vi "13.4.2 AutoROI.vi"(8 "ErrI":errorcluster) -> (0 "ErrO":errorcluster)   [LabVIEW 2016]
uses:
  <vilib>/vision/Image Controls.llb/IMAQ Image.ctl
  <vilib>/vision/Measure.llb/Edge Options.ctl
  <vilib>/vision/Measure.llb/Edge Polarity.ctl
  <vilib>/vision/NI_Vision_Development_Module.lvlib
panel:
  out "Coordinate System":T1 {"Measurement System"."Axis Reference" items=["Direct", "Indirect"]; "Measurement System"."Angle (deg)" format="%.2f"; "Measurement System"."Origin"."Y" format="%.2f"; "Measurement System"."Origin"."X" format="%.2f"; "Reference System"."Axis Reference" items=["Direct", "Indirect"]; "Reference System"."Angle (deg)" format="%.2f"; "Reference System"."Origin"."Y" format="%.2f"; "Reference System"."Origin"."X" format="%.2f"}
  out "Distance":sgl format="%.2f"
  out "Image":T2(plugin-control)
  in  "Next":bool
  in  "Exit":bool
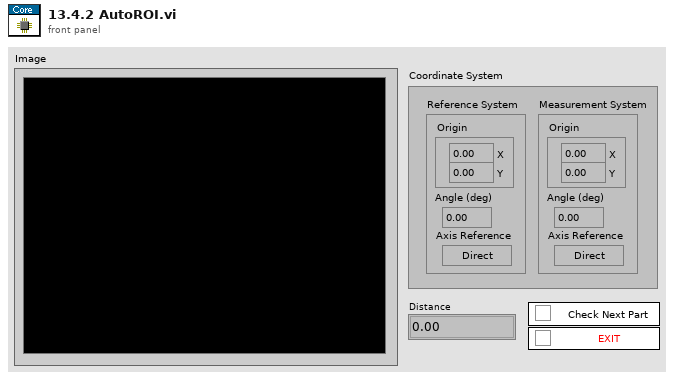
[diagram p1: front panel]
types:
  T1 = typedef "IMAQ Coordinate System" = cluster{"Reference System":cluster{"Origin":cluster{"X":sgl, "Y":sgl}, "Angle (deg)":sgl, "Axis Reference":u32}, "Measurement System":cluster{"Origin":cluster{"X":sgl, "Y":sgl}, "Angle (deg)":sgl, "Axis Reference":u32}}
  T2 = typedef "IMAQ Image.ctl" = refnum<image>
  T3 = typedef "IMAQ Rectangle" = cluster{"Left":i32, "Top":i32, "Right":i32, "Bottom":i32, "Rotation":dbl}
  T4 = cluster{"Contrast":i32, "Filter width":i32, "Steepness":i32, "Subsampling Ratio":u32, "Show Search Area":bool, "Show Search Lines":bool, "Show Edges Found":bool, "Show Result":bool}
  T5 = cluster{"Src":T2, "Dst":T2, "Parts":string[], "RefCoord":T1, "MsrCoord":T1, "MsrROI":T3}
  T6 = typedef "Edge Options.ctl" = cluster{"Edge Polarity":T7, "Kernel Size":u32, "Width":u32, "Minimum Edge Strength":sgl, "Interpolation Type":enum32{"Zero Order", "Bilinear", "Quadratic", "Cubic", "Bilinear Fixed"}, "Data Processing Method":enum32{"Average", "Median"}}
  T7 = typedef "Edge Polarity.ctl" = u32
  T8 = cluster{"Direction":u16, "Edge Options":T6, "Show Search Area":bool, "Show Search Lines":bool, "Show Edges Found":bool, "Show Result":bool, "Search Area Color":u32, "Search Lines Color":u32, "Edge Locations Color":u32, "Result Color":u32, "Overlay Group Name":string}
  T9 = typedef "ROI Descriptor" = cluster{"Global Rectangle":i32[], "Contours":cluster{"ID":enum32{"External", "Internal"}, "Type":u32, "Coordinates":i32[]}[]}
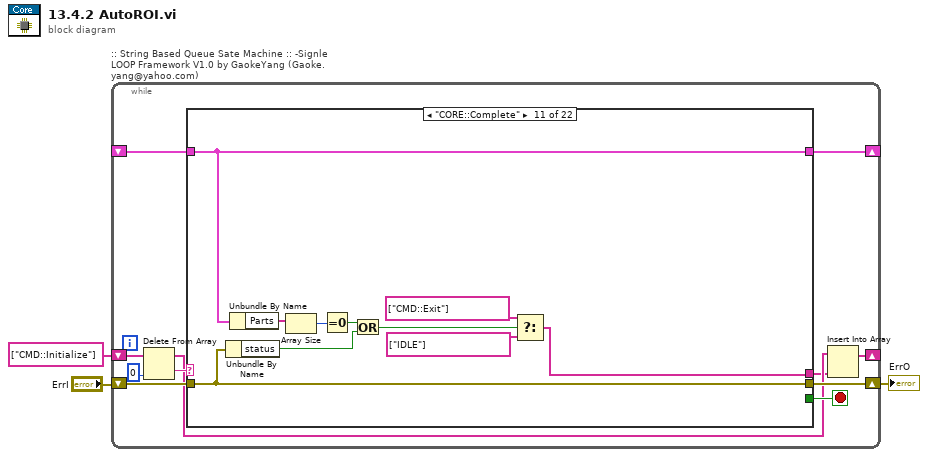
[diagram p0: block diagram]
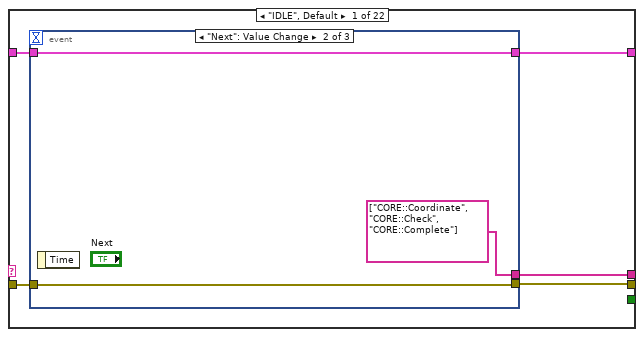
[diagram p2: hidden frame]
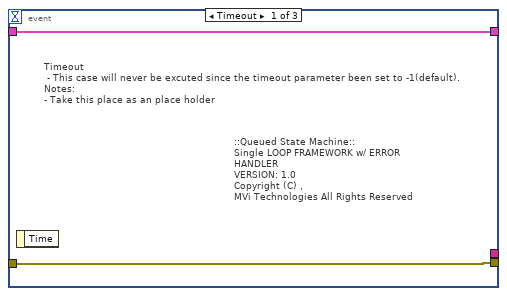
[diagram p3: hidden frame]
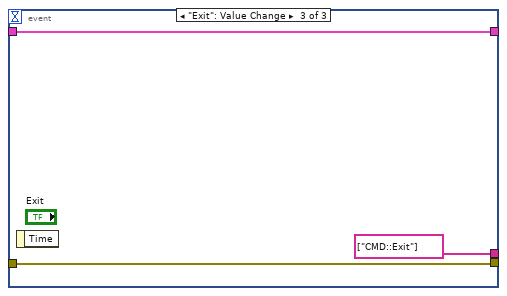
[diagram p4: hidden frame]
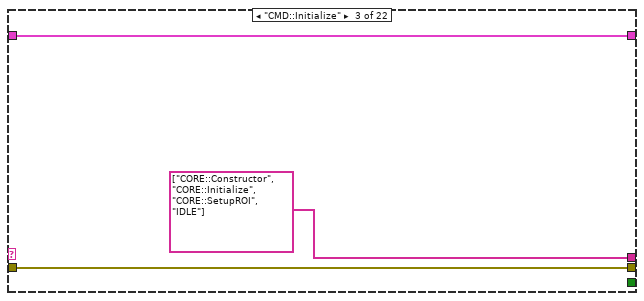
[diagram p6: hidden frame]
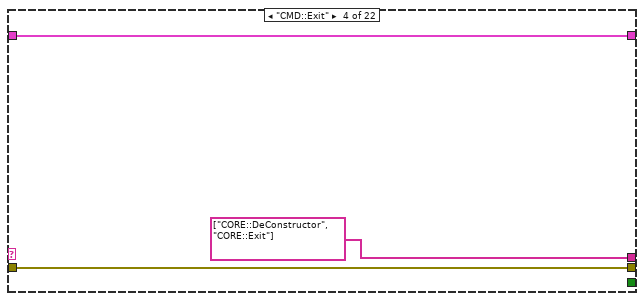
[diagram p7: hidden frame]
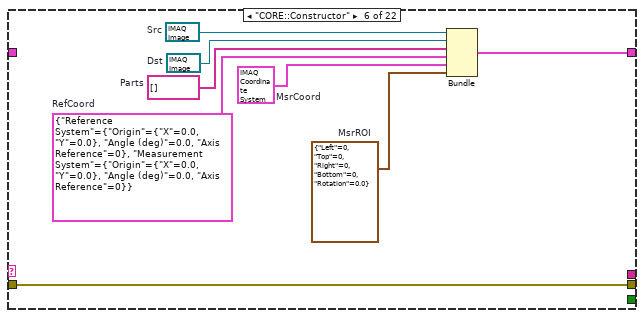
[diagram p9: hidden frame]
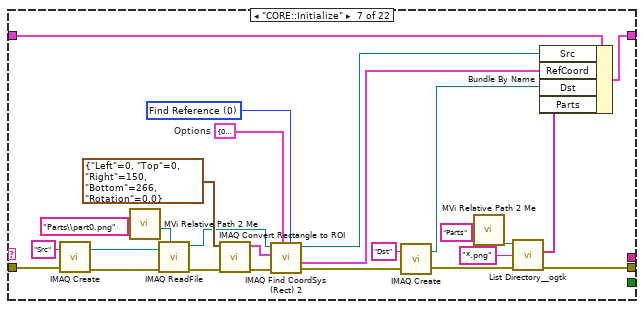
[diagram p10: hidden frame]
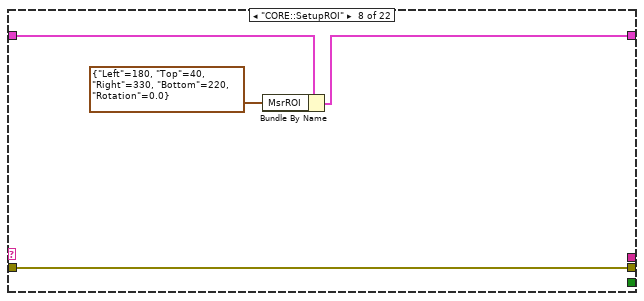
[diagram p11: hidden frame]
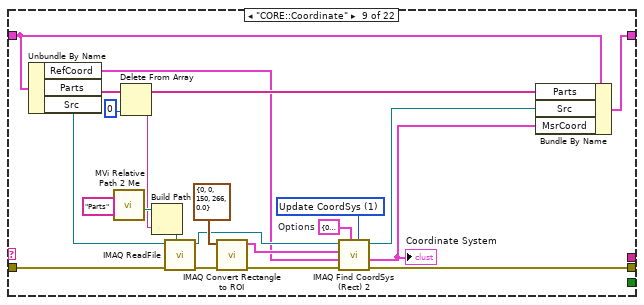
[diagram p12: hidden frame]
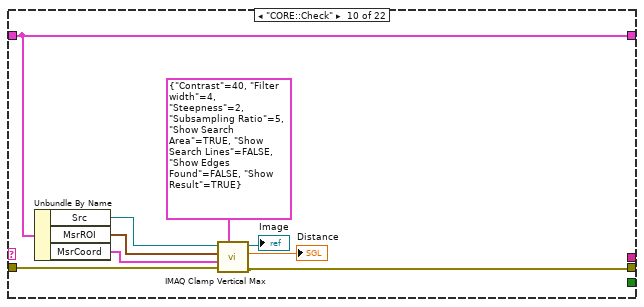
[diagram p13: hidden frame]
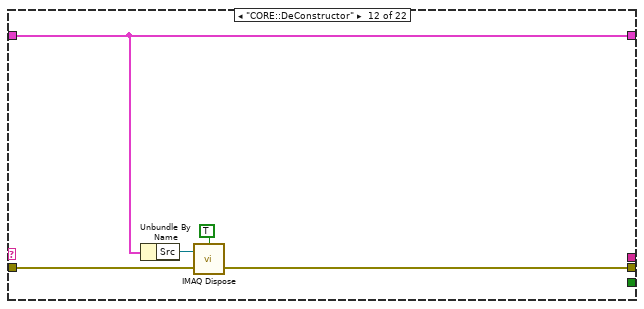
[diagram p14: hidden frame]
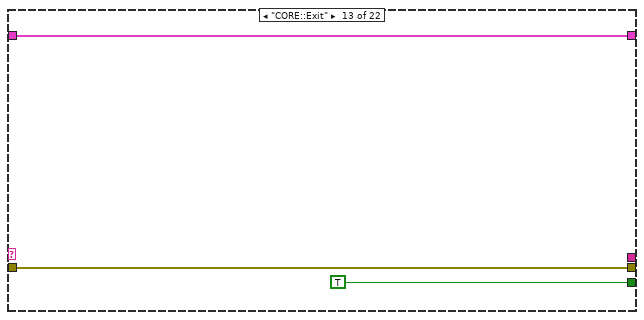
[diagram p15: hidden frame]
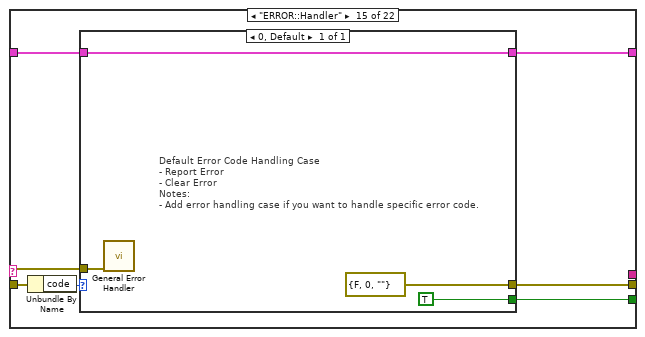
[diagram p17: hidden frame]
diagram:
  n1 = while ":: String Based Queue Sate Machine :: -Signle LOOP Framework V1.0 by GaokeYang (Gaoke.yang@yahoo.com)" {
    shift-right: [w11] -> w3
    shift-left: "ErrI" -> [w9]
    shift-right: [w13] -> _
    shift-left: _ -> [w12]
    shift-right: [w4] -> _
    shift-left: string[] ["CMD::Initialize"] -> [w10]
    stop <- w14 stop-if-true
    n2 = Delete From Array(array=w10, index=0) -> (deleted portion=w8:string, array with subset deleted=w6:string[])  [unwired: 1 in]
    n3 = case shown="\"CORE::Complete\"" w8 {
      tunnel: [w18 w29 w31 w34 w37 w44 w60 w72 w79 w104 w112 w120 w122 w126 w129 w137 w139 w141 w144 w146 w148 w149] -> w11
      tunnel: [_ _ _ _ _ _ _ _ _ _ _ _ TRUE _ w128 _ _ _ _ _ _ _] -> w14
      tunnel: w9 -> [w19 w29 w31 w34 w37 w44 w64 w72 w92 w105 w112 w121 w122 w126 w127 w137 w139 w141 w144 w146 w148 w149]
      tunnel: [w16 w28 w32 w35 w36 w45 w68 w75 w89 w106 w113 w119 w123 w125 w130 w138 w140 w142 w143 w145 w147 w150] -> w13
      tunnel: w12 -> [w17 w28 w32 w35 w36 _ w69 w74 w90 w106 w113 w119 w123 w125 w131 w138 w140 w142 w143 w145 w147 w150]
      tunnel: [w15 _ string[] ["CORE::Constructor", "CORE::Initialize", "CORE::SetupROI", "IDLE"] string[] ["CORE::DeConstructor", "CORE::Exit"] _ _ _ _ _ _ w114 _ _ _ _ _ _ _ _ _ _ _] -> w5
      frame "IDLE", Default {
        n4 = event shown="[1] \"Next\": Value Change" {
          selector: _ -> [_ _ _]
          dyn-events: _ -> [_ _ _]
          timeout: _ -> [_ _ _]
          tunnel: [w21 w24 w27] -> w18
          tunnel: w19 -> [w21 w24 w27]
          tunnel: [w20 w23 w26] -> w16
          tunnel: w17 -> [w20 w23 w26]
          tunnel: [_ string[] ["CORE::Coordinate", "CORE::Check", "CORE::Complete"] string[] ["CMD::Exit"]] -> w15
          event Timeout {
            # "Timeout\n - This case will never be excuted since the timeout parameter been set to -1(default).\nNotes:\n- Take this place as an place holder"
            # "::Queued State Machine::\nSingle LOOP FRAMEWORK w/ ERROR HANDLER\nVERSION: 1.0\nCopyright (C) ,\nMVi Technologies All Rights Reserved"
            n5 = event-data() -> ()  [unwired: 1 in, 1 out]
          }
          event "Next": Value Change {
            n6 = event-data() -> ()  [unwired: 1 in, 1 out]
          }
          event "Exit": Value Change {
            n7 = event-data() -> ()  [unwired: 1 in, 1 out]
          }
        }
      }
      frame "-------- Commands ---------" {
      }
      frame "CMD::Initialize" {
      }
      frame "CMD::Exit" {
      }
      frame "------------ Core ------------" {
      }
      frame "CORE::Constructor" {
        w38 = T3 {"Left"=0, "Top"=0, "Right"=0, "Bottom"=0, "Rotation"=0.0}  # MsrROI
        w39 = T1 {"Reference System"={"Origin"={"X"=0.0, "Y"=0.0}, "Angle (deg)"=0.0, "Axis Reference"=0}, "Measurement System"={"Origin"={"X"=0.0, "Y"=0.0}, "Angle (deg)"=0.0, "Axis Reference"=0}}  # MsrCoord
        w40 = T1 {"Reference System"={"Origin"={"X"=0.0, "Y"=0.0}, "Angle (deg)"=0.0, "Axis Reference"=0}, "Measurement System"={"Origin"={"X"=0.0, "Y"=0.0}, "Angle (deg)"=0.0, "Axis Reference"=0}}  # RefCoord
        w43 = T2 refnum  # Dst
        w42 = string[] []  # Parts
        w41 = T2 refnum  # Src
        n8 = Bundle("Src"=w41, "Dst"=w43, "Parts"=w42, "RefCoord"=w40, "MsrCoord"=w39, "MsrROI"=w38) -> (w45:T5)  [unwired: 1 in]
      }
      frame "CORE::Initialize" {
        w46 = u16 0 items=["Find Reference", "Update CoordSys"] ("Mode")
        w47 = T8 {"Direction"=0, "Edge Options"={"Edge Polarity"=0, "Kernel Size"=3, "Width"=3, "Minimum Edge Strength"=10.0, "Interpolation Type"=enum."Bilinear Fixed", "Data Processing Method"=enum."Average"}, "Show Search Area"=FALSE, "Show Search Lines"=FALSE, "Show Edges Found"=FALSE, "Show Result"=TRUE, "Search Area Color"=65280, "Search Lines Color"=255, "Edge Locations Color"=16776960, "Result Color"=16711680, "Overlay Group Name"=""}  # Options
        n9 = call "IMAQ Create"("Image Name"="Src", "error in (no error)"=w64) -> ("Src"=w67:T2, "error out"=w65:errorcluster)  [unwired: 3 in]
        n10 = call "MVi Relative Path 2 Me.vi"("Relative Path"="Parts\\part0.png" ("name or relative path")) -> ("Appended Dir"=w66:path)  [unwired: 5 in, 1 out]
        n11 = call "IMAQ ReadFile"("File Path"=w66, "error in (no error)"=w65, "Image"=w67) -> ("error out"=w57:errorcluster, "Image Out"=w54:T2)  [unwired: 4 in, 3 out]
        n12 = call "IMAQ Convert Rectangle to ROI"("error in (no error)"=w57, "Rectangle"=T3 {"Left"=0, "Top"=0, "Right"=150, "Bottom"=266, "Rotation"=0.0}) -> ("error out"=w55:errorcluster, "ROI Descriptor"=w53:T9)  [unwired: 7 in]
        n13 = call "IMAQ Find CoordSys (Rect) 2"("Mode"=w46, "Options"=w47, "error in (no error)"=w55, "ROI Descriptor"=w53, "Image"=w54) -> ("error out"=w52:errorcluster, "Coordinate System Out"=w49:T1, "Image Out"=w51:T2)  [unwired: 2 in, 2 out]
        n14 = call "IMAQ Create"("Image Name"="Dst", "error in (no error)"=w52) -> ("Src"=w50:T2, "error out"=w58:errorcluster)  [unwired: 3 in]
        n15 = call "MVi Relative Path 2 Me.vi"("Relative Path"="Parts" ("name or relative path")) -> ("Appended Dir"=w62:path)  [unwired: 5 in, 1 out]
        n16 = call "List Directory__ogtk.vi"("error in (no error)"=w58, "pattern"="*.png", "directory path"=w62) -> ("error out"=w60:errorcluster, "file names"=w48:string[])  [unwired: 1 in, 2 out]
        n17 = Bundle By Name(cluster=w69, "Src"=w51, "RefCoord"=w49, "Dst"=w50, "Parts"=w48) -> (w68:T5)
      }
      frame "CORE::SetupROI" {
        n18 = Bundle By Name(cluster=w74, "MsrROI"=T3 {"Left"=180, "Top"=40, "Right"=330, "Bottom"=220, "Rotation"=0.0} ("Rectangle")) -> (w75:T5)
      }
      frame "CORE::Coordinate" {
        w76 = T8 {"Direction"=0, "Edge Options"={"Edge Polarity"=0, "Kernel Size"=3, "Width"=3, "Minimum Edge Strength"=10.0, "Interpolation Type"=enum."Bilinear Fixed", "Data Processing Method"=enum."Average"}, "Show Search Area"=FALSE, "Show Search Lines"=FALSE, "Show Edges Found"=FALSE, "Show Result"=TRUE, "Search Area Color"=65280, "Search Lines Color"=255, "Edge Locations Color"=16776960, "Result Color"=16711680, "Overlay Group Name"=""}  # Options
        w88 = u16 1 items=["Find Reference", "Update CoordSys"] ("Mode")
        n19 = Unbundle By Name(w90) -> ("RefCoord"=w80:T1, "Parts"=w87:string[], "Src"=w86:T2)
        n20 = call "MVi Relative Path 2 Me.vi"("Relative Path"="Parts" ("name or relative path")) -> ("Appended Dir"=w96:path)  [unwired: 5 in, 1 out]
        n21 = Delete From Array(array=w87, index=0) -> (deleted portion=w94:string, array with subset deleted=w91:string[])  [unwired: 1 in]
        n22 = Build Path(base path=w96, name or relative path=w94) -> (appended path=w93:path)
        n23 = call "IMAQ ReadFile"("File Path"=w93, "error in (no error)"=w92, "Image"=w86) -> ("error out"=w85:errorcluster, "Image Out"=w81:T2)  [unwired: 4 in, 3 out]
        n24 = call "IMAQ Convert Rectangle to ROI"("error in (no error)"=w85, "Rectangle"=T3 {"Left"=0, "Top"=0, "Right"=150, "Bottom"=266, "Rotation"=0.0}) -> ("error out"=w84:errorcluster, "ROI Descriptor"=w82:T9)  [unwired: 7 in]
        n25 = call "IMAQ Find CoordSys (Rect) 2"("Mode"=w88, "Options"=w76, "error in (no error)"=w84, "Coordinate System In"=w80, "ROI Descriptor"=w82, "Image"=w81) -> ("error out"=w79:errorcluster, "Coordinate System Out"=w77:T1, "Image Out"=w78:T2)  [unwired: 1 in, 2 out]
        "Coordinate System" <- w77
        n26 = Bundle By Name(cluster=w90, "Parts"=w91, "Src"=w78, "MsrCoord"=w77) -> (w89:T5)
      }
      frame "CORE::Check" {
        n27 = Unbundle By Name(w106) -> ("Src"=w101:T2, "MsrROI"=w102:T3, "MsrCoord"=w100:T1)
        n28 = call "IMAQ Clamp Vertical Max"("Settings"=T4 {"Contrast"=40, "Filter width"=4, "Steepness"=2, "Subsampling Ratio"=5, "Show Search Area"=TRUE, "Show Search Lines"=FALSE, "Show Edges Found"=FALSE, "Show Result"=TRUE}, "error in (no error)"=w105, "Coordinate System"=w100, "Rectangle"=w102, "Image"=w101) -> ("error out"=w104:errorcluster, "Distance"=→"Distance":sgl, "Image Out"=→"Image":T2)  [unwired: 2 in, 2 out]
      }
      frame "CORE::Complete" {
        n29 = Unbundle By Name(w112) -> ("status"=w108:bool)
        n30 = Unbundle By Name(w113) -> ("Parts"=w111:string[])
        n31 = Array Size(array=w111) -> (size(s)=w110:i32)
        n32 = Equal To 0?(x=w110) -> (x = 0?=w109:bool)
        n33 = Or(x=w109, y=w108) -> (x .or. y?=w107:bool)
        n34 = Select(t=string[] ["CMD::Exit"], s=w107, f=string[] ["IDLE"]) -> (s? t:f=w114:string[])
      }
      frame "CORE::DeConstructor" {
        n35 = Unbundle By Name(w119) -> ("Src"=w118:T2)
        n36 = call "IMAQ Dispose"("All Images? (No)"=TRUE, "Image"=w118, "error in (no error)"=w121) -> ("error out"=w120:errorcluster)  [unwired: 3 in]
      }
      frame "CORE::Exit" {
      }
      frame "-------- Error Handle--------" {
      }
      frame "ERROR::Handler" {
        n37 = Unbundle By Name(w127) -> ("code"=w132:i32)
        n38 = case shown="0, Default" w132 {
          tunnel: [w136] -> w130
          tunnel: w131 -> [w136]
          tunnel: [errorcluster {"status"=FALSE, "code"=0, "source"=""} ("error out")] -> w129
          tunnel: [TRUE] -> w128
          tunnel: w127 -> [w134]
          frame 0, Default {
            # "Default Error Code Handling Case\n- Report Error\n- Clear Error \nNotes:\n- Add error handling case if you want to handle specific error code."
            n39 = call <vilib>:"General Error Handler.vi"("error in (no error)"=w134) -> ()  [unwired: 10 in, 5 out]
          }
        }
      }
      frame "------------  GUI  ------------" {
      }
      frame "GUI::Initialize" {
      }
      frame "GUI::SetCusor" {
      }
      frame "GUI::SetMenu" {
      }
      frame "------------ USER -----------" {
      }
      frame "USER::Case1" {
      }
      frame "USER::Case2" {
      }
    }
    n40 = Insert Into Array(array=w6, new element=w5) -> (w4:string[])  [unwired: 1 in]
  }
  "ErrO" <- w3
